vi "Car3UDPmsg_parse.vi"(11 "error in (no error)":errorcluster) -> (15 "error out":errorcluster)   [LabVIEW 2020]
panel:
  # "Parse a CARIBIC-3 (A350) UDP message.\n\nInputs:\n- byte string\n\nOutput:\n- byte string\n- sender address IPv4 and port\n- receiver address IPv4 and port\n- message length (n bytes)\n- message composition timestamp\n- message type\n- message data\n- message checksum\n\n\nDependencies (besides standard lib):\n- checksum calculation vi\n\nLabVIEW version:\n- written with LV 2020 f1"
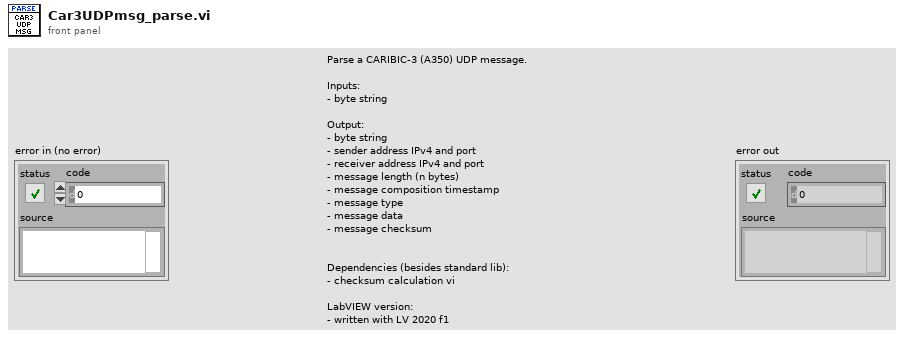
[diagram p1: front panel]
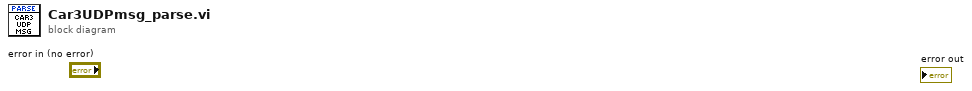
[diagram p0: block diagram]
diagram:
